vi "CheckIfConnectorPanesMatch.vi"(8 "error in (no error)":errorcluster, 9 "terminal subset acceptable (false)":bool, 10 "actual connector pane vi":path, 11 "expected connector pane vi":path) -> (0 "error out":errorcluster, 1 "mismatch explanation":string, 3 "connector panes match":bool)   [LabVIEW 2015, in "VeriStandTestUtilities.lvlib"]
uses:
  VeriStandTestUtilities.lvlib
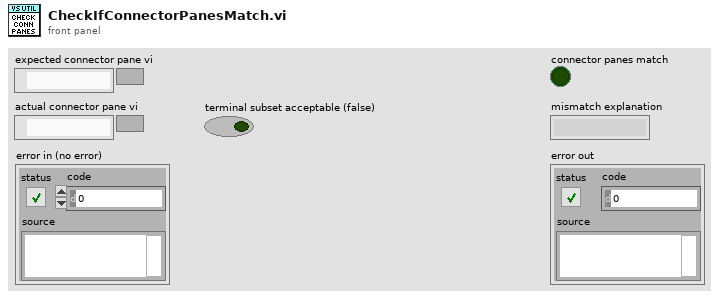
[diagram p1: front panel]
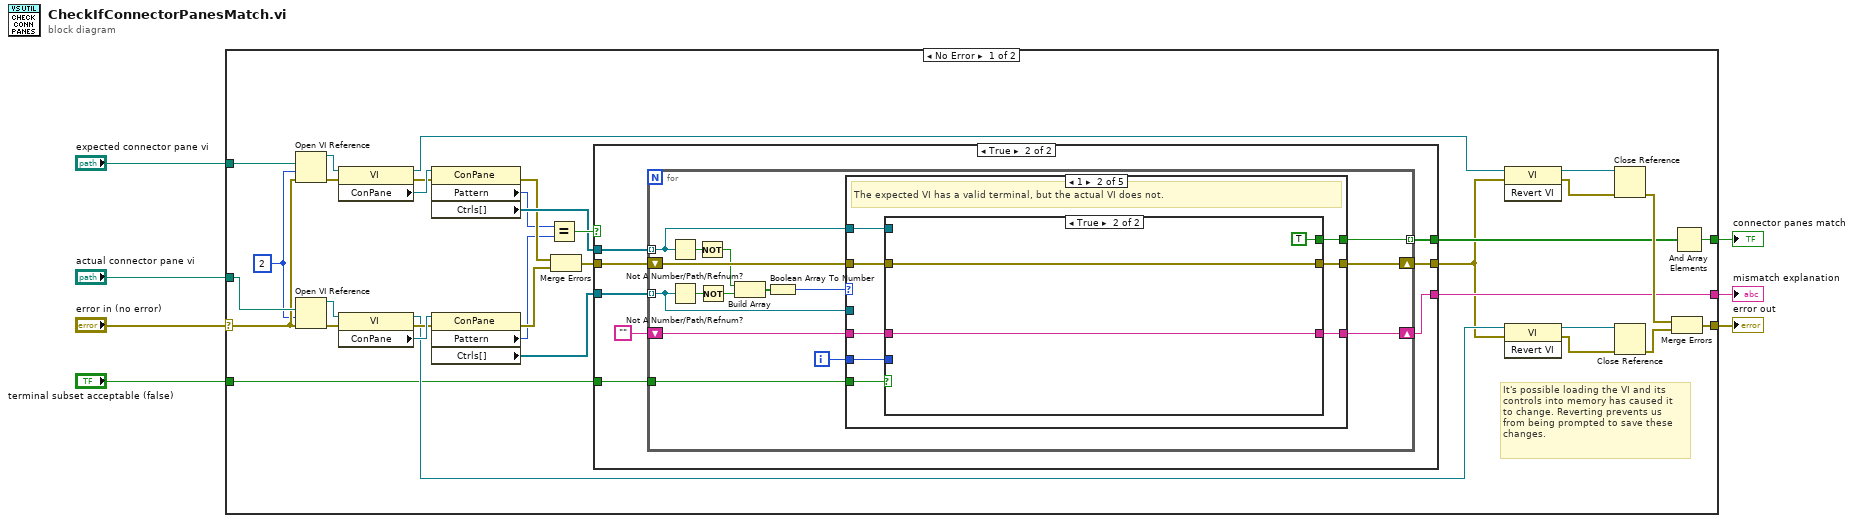
[diagram p0: block diagram]
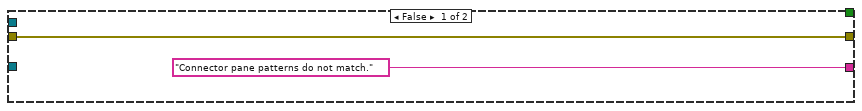
[diagram p2: hidden frame]
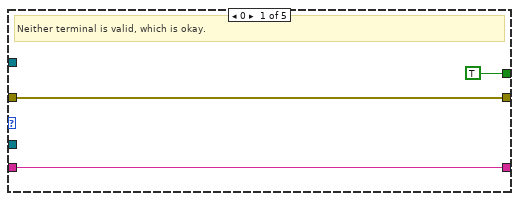
[diagram p3: hidden frame]
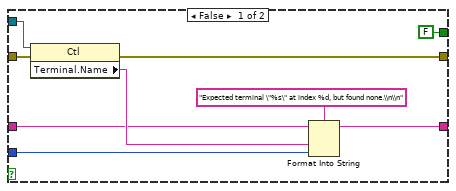
[diagram p4: hidden frame]
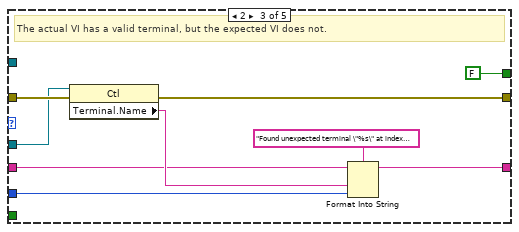
[diagram p5: hidden frame]
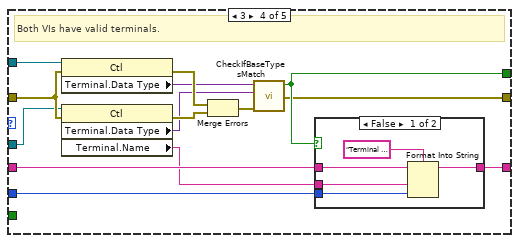
[diagram p6: hidden frame]
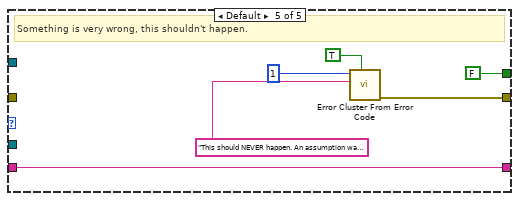
[diagram p8: hidden frame]
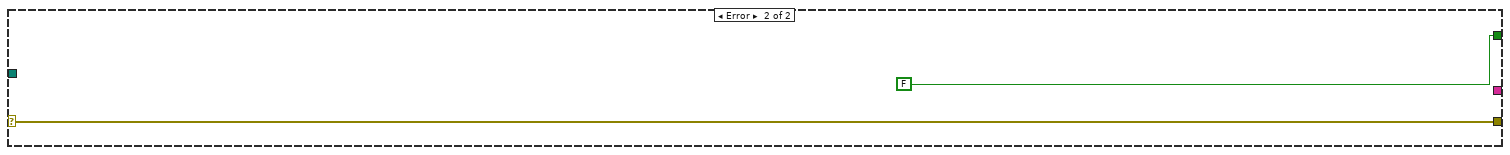
[diagram p9: hidden frame]
diagram:
  n1 = case shown="No Error" "error in (no error)" {
    selector: "error in (no error)" -> [w33 w126]
    tunnel: "actual connector pane vi" -> [w41 _]
    tunnel: "expected connector pane vi" -> [w35 _]
    tunnel: [w22 w126] -> w4
    tunnel: [w21 FALSE] -> w3
    tunnel: [w17 _] -> w2
    tunnel: "terminal subset acceptable (false)" -> [w8 _]
    frame No Error {
      w16 = 2 ("options")
      # "It's possible loading the VI and its\ncontrols into memory has caused it\nto change. Reverting prevents us\nfrom being prompted to save these\nchanges."
      n2 = Open VI Reference(vi path=w35, options=w16, error in (no error)=w33) -> (vi reference=w36:refnum<vi>, error out=w37:errorcluster)  [unwired: 3 in]
      n3 = Open VI Reference(vi path=w41, options=w16, error in (no error)=w33) -> (vi reference=w40:refnum<vi>, error out=w39:errorcluster)  [unwired: 3 in]
      n4 = property class="VI"(reference=w36, error in=w37) -> (reference out=w9:refnum<vi>, error out=w28:errorcluster, "ConPane"=w34:refnum<vi>)
      n5 = property class="VI"(reference=w40, error in=w39) -> (reference out=w14:refnum<vi>, error out=w29:errorcluster, "ConPane"=w38:refnum<vi>)
      n6 = property class="ConPane"(reference=w34, error in=w28) -> (error out=w27:errorcluster, "Pattern"=w19:u32, "Ctrls[]"=w31:refnum<vi>[])  [unwired: 1 out]
      n7 = property class="ConPane"(reference=w38, error in=w29) -> (error out=w26:errorcluster, "Pattern"=w20:u32, "Ctrls[]"=w30:refnum<vi>[])  [unwired: 1 out]
      n8 = Equal?(x=w19, y=w20) -> (x = y?=w32:bool)
      n9 = Merge Errors(w27, w26) -> (w25:errorcluster)
      n10 = case shown="True" w32 {
        tunnel: w30 -> [_ w51]
        tunnel: w31 -> [_ w50]
        tunnel: w25 -> [w43 w49]
        tunnel: [w43 w48] -> w11
        tunnel: [_ w47] -> w18
        tunnel: ["Connector pane patterns do not match." w45] -> w17
        tunnel: w8 -> [_ w44]
        frame False {
        }
        frame True {
          n11 = for {
            tunnel: w51 -> [w54] mode=indexing
            tunnel: w50 -> [w55] mode=indexing
            tunnel: [w56] -> w47 mode=indexing
            shift-right: [w61] -> w48
            shift-left: w49 -> [w62]
            shift-right: [w59] -> w45
            shift-left: "" -> [w60]
            tunnel: w44 -> [w52]
            i -> [w53]
            n12 = Not A Number/Path/Refnum?(number/path/refnum=w55) -> (NaN/Path/Refnum?=w66:bool)
            n13 = Not A Number/Path/Refnum?(number/path/refnum=w54) -> (NaN/Path/Refnum?=w65:bool)
            n14 = Not(x=w66) -> (.not. x?=w58:bool)
            n15 = Not(x=w65) -> (.not. x?=w57:bool)
            n16 = Build Array(w58, w57) -> (w64:bool[])
            n17 = Boolean Array To Number(Boolean array=w64) -> (number=w63:u32)
            n18 = case shown="1" w63 {
              tunnel: w62 -> [w69 w76 w95 w109 _]
              tunnel: [w69 w75 w96 w99 w124] -> w61
              tunnel: w60 -> [w68 w74 w92 w108 w122]
              tunnel: [w68 w73 w91 w107 w122] -> w59
              tunnel: [TRUE w71 FALSE w101 FALSE] -> w56
              tunnel: w55 -> [_ w77 _ w105 _]
              tunnel: w54 -> [_ _ w94 w104 _]
              tunnel: w53 -> [_ w72 w93 w106 _]
              tunnel: w52 -> [_ w70 _ _ _]
              frame 0 {
                # "Neither terminal is valid, which is okay."
              }
              frame 1 {
                # "The expected VI has a valid terminal, but the actual VI does not."
                n19 = case shown="True" w70 {
                  tunnel: w77 -> [w85 _]
                  tunnel: w76 -> [w84 w88]
                  tunnel: [w83 w88] -> w75
                  tunnel: w74 -> [w82 w87]
                  tunnel: [w81 w87] -> w73
                  tunnel: w72 -> [w79 _]
                  tunnel: [FALSE TRUE] -> w71
                  frame False {
                    n20 = property class="Ctl"(reference=w85, error in=w84) -> (error out=w83:errorcluster, "Terminal.Name"=w86:string)  [unwired: 1 out]
                    n21 = Format Into String(format string="Expected terminal \"%s\" at index %d, but found none.\\n\\n", initial string=w82, w86, w79) -> (resulting string=w81:string)  [unwired: 1 in, 1 out]
                  }
                  frame True {
                  }
                }
              }
              frame 2 {
                # "The actual VI has a valid terminal, but the expected VI does not."
                n22 = property class="Ctl"(reference=w94, error in=w95) -> (error out=w96:errorcluster, "Terminal.Name"=w98:string)  [unwired: 1 out]
                n23 = Format Into String(format string="Found unexpected terminal \"%s\" at index %d, expected none.\\n\\n", initial string=w92, w98, w93) -> (resulting string=w91:string)  [unwired: 1 in, 1 out]
              }
              frame 3 {
                # "Both VIs have valid terminals."
                n24 = property class="Ctl"(reference=w105, error in=w109) -> (error out=w112:errorcluster, "Terminal.Data Type"=w110:variant)  [unwired: 1 out]
                n25 = property class="Ctl"(reference=w104, error in=w109) -> (error out=w111:errorcluster, "Terminal.Data Type"=w102:variant, "Terminal.Name"=w103:string)  [unwired: 1 out]
                n26 = Merge Errors(w112, w111) -> (w100:errorcluster)
                n27 = call "CheckIfBaseTypesMatch.vi"("error in (no error)"=w100, "Actual data type"=w102, "Expected data type"=w110) -> ("error out"=w99:errorcluster, "types match"=w101:bool)  [unwired: 7 in]
                n28 = case shown="False" w101 {
                  tunnel: [w117 w118] -> w107
                  tunnel: w108 -> [w114 w118]
                  tunnel: w106 -> [w115 _]
                  tunnel: w103 -> [w113 _]
                  frame False {
                    n29 = Format Into String(format string="Terminal \"%s\" at index %d does not have expected type.\\n\\n", initial string=w114, w113, w115) -> (resulting string=w117:string)  [unwired: 1 in, 1 out]
                  }
                  frame True {
                  }
                }
              }
              frame Default {
                # "Something is very wrong, this shouldn't happen."
                n30 = call <vilib>:"Error Cluster From Error Code.vi"("show call chain? (False)"=TRUE, "error message (\"\")"="This should NEVER happen. An assumption was made that exactly two boolean statements were being checked together; either this has been changed, or a case has been removed and not handled properly." ("error message (\"\")"), "error code (0)"=1) -> ("error out"=w124:errorcluster)  [unwired: 6 in]
              }
            }
          }
        }
      }
      n31 = invoke class="VI" method="Revert VI"(reference=w9, error in=w11) -> (reference out=w10:refnum<vi>, error out=w12:errorcluster)  [unwired: 1 in, 1 out]
      n32 = invoke class="VI" method="Revert VI"(reference=w14, error in=w11) -> (reference out=w15:refnum<vi>, error out=w13:errorcluster)  [unwired: 1 in, 1 out]
      n33 = Close Reference(reference=w10, error in (no error)=w12) -> (error out=w23:errorcluster)
      n34 = Close Reference(reference=w15, error in (no error)=w13) -> (error out=w24:errorcluster)
      n35 = Merge Errors(w23, w24) -> (w22:errorcluster)
      n36 = And Array Elements(Boolean array=w18) -> (logical AND=w21:bool)
    }
    frame Error {
    }
  }
  "error out" <- w4
  "connector panes match" <- w3
  "mismatch explanation" <- w2
